vi "Module Queue FGV.vi"(8 "Error in":errorcluster, 9 "Queue name":string, 10 "Action":T1=enum."Destroy") -> (0 "Error out":errorcluster, 3 "Queue ref":refnum<queue>)   [LabVIEW 2018, in "Error Handler.lvlib"]
doc: "Used for module queue admin."
uses:
  Error Handler.lvlib
  ctl/Module Queue - Action.ctl
  ctl/Module - Message.ctl
  ctl/Module - State.ctl
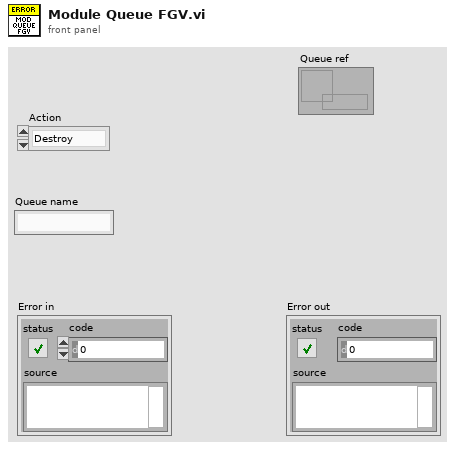
[diagram p1: front panel]
types:
  T1 = typedef "Error Handler.lvlib/Module Queue - Action.ctl" = enum16{"Create", "Get", "Destroy"}
  T2 = typedef "Error Handler.lvlib/Module - Message.ctl" = cluster{"State":T3, "Data":variant}
  T3 = typedef "Error Handler.lvlib/Module - State.ctl" = enum16{"Init", "Idle", "Error", "Close", "Handle External Error", "Log Error"}
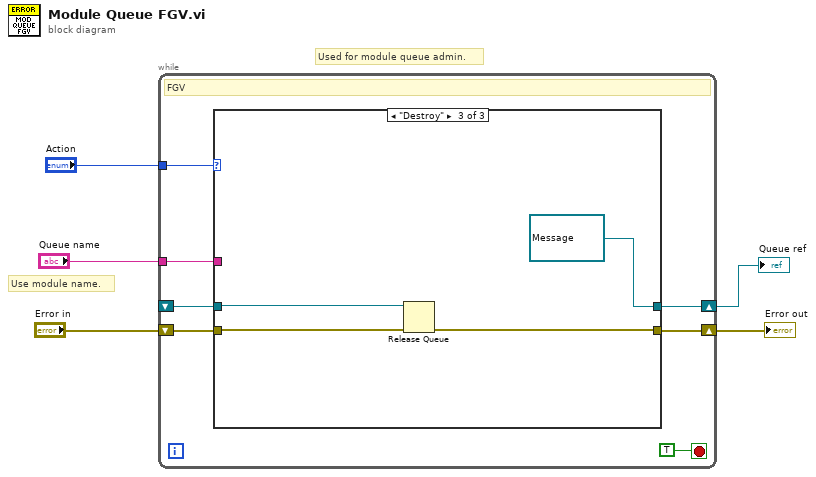
[diagram p0: block diagram]
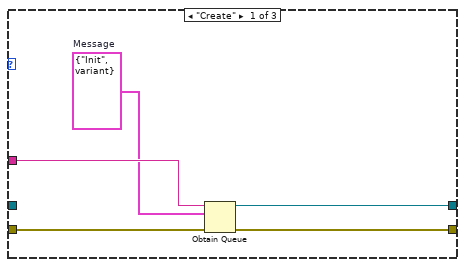
[diagram p2: hidden frame]
diagram:
  # "Used for module queue admin."
  # "Use module name."
  n1 = while {
    tunnel: "Action" -> [w11]
    shift-right: [w10] -> w1
    shift-left: _ -> [w6]
    shift-right: [w9] -> w4
    shift-left: "Error in" -> [w8]
    tunnel: "Queue name" -> [w7]
    stop <- TRUE stop-if-true
    # "FGV"
    n2 = case shown="\"Destroy\"" w11 {
      tunnel: [w17 w18 refnum<queue> refnum ("queue out")] -> w10
      tunnel: [w16 w19 w21] -> w9
      tunnel: w8 -> [w15 w19 w22]
      tunnel: w7 -> [w14 _ _]
      tunnel: w6 -> [_ w18 w23]
      frame "Create" {
        w13 = T2 {"State"=enum."Init", "Data"=variant}  # Message
        n3 = Obtain Queue(name (unnamed)=w14, element data type=w13, error in (no error)=w15) -> (queue out=w17:refnum<queue>, error out=w16:errorcluster)  [unwired: 2 in, 1 out]
      }
      frame "Get", Default {
      }
      frame "Destroy" {
        n4 = Release Queue(queue=w23, error in (no error)=w22) -> (error out=w21:errorcluster)  [unwired: 1 in, 2 out]
      }
    }
  }
  "Error out" <- w4
  "Queue ref" <- w1
